vi "seq_test.vi"() -> ()   [LabVIEW 2015]
uses:
  BERTTA.dll
panel:
  out "Waveform Chart 2":dynamicdata(graph)
  out "Waveform Chart":dynamicdata(graph)
  in  "Boolean":bool
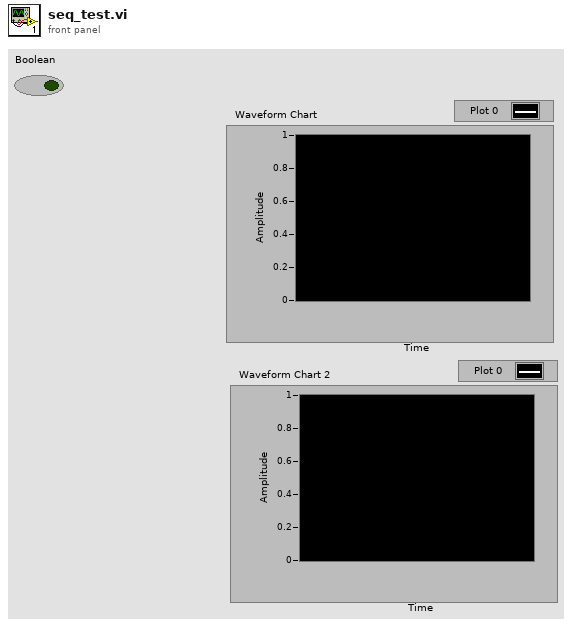
[diagram p1: front panel]
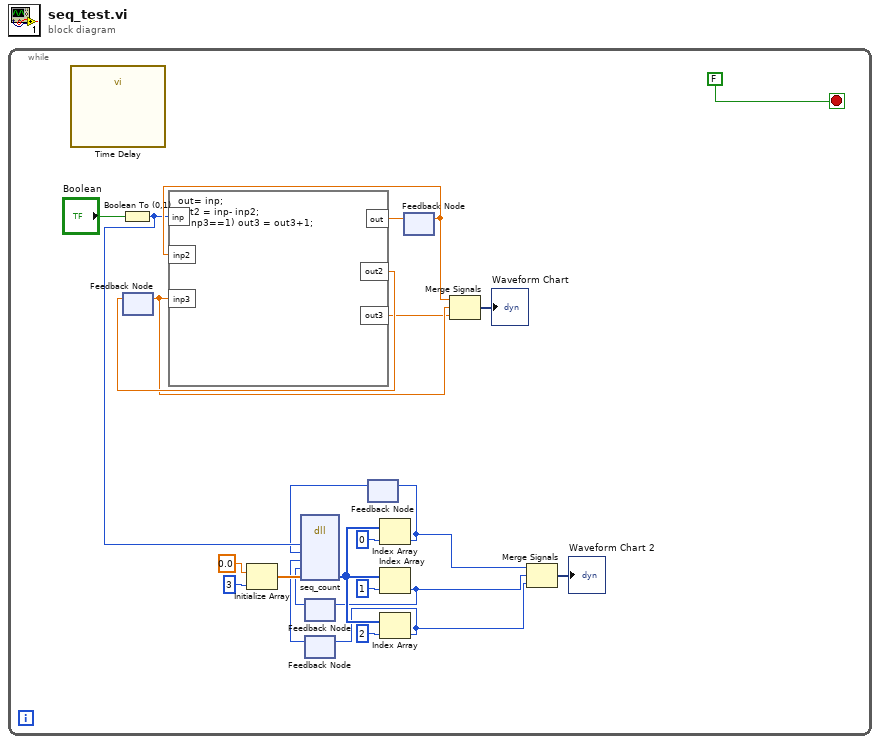
[diagram p0: block diagram]
diagram:
  n1 = while {
    stop <- FALSE stop-if-true
    n2 = call "Time Delay"() -> ()  [unwired: 11 in, 1 out]
    n3 = Boolean To (0,1)(Boolean="Boolean") -> (0, 1=w15:i16)
    n4 = feedback #1() -> (w17:dbl)  [unwired: 1 in]
    n5 = Initialize Array(0.0 ("element"), 3 ("dimension size")) -> (w14:dbl[])
    n6 = feedback #2() -> (w5:i32)  [unwired: 1 in]
    n7 = feedback #3() -> (w7:i32)  [unwired: 1 in]
    n8 = feedback #4() -> (w6:i32)  [unwired: 1 in]
    n9 = dll-call lib="C:/Users/xlaraser/Documents/Visual Studio 2017/Projects/Bertta/BERTTA/Debug/BERTTA.dll" fn="seq_count"("in1"=w15, "in2"=w6, "in3"=w7, "in4"=w5, "params"=w14) -> ("params"=w8:i32[])  [unwired: 8 in, 2 out]
    n10 = Index Array(array=w8, index=0) -> (element=w3:i32)
    n11 = feedback-in #4(w3) -> ()
    n12 = Index Array(array=w8, index=1) -> (element=w2:i32)
    n13 = feedback-in #2(w2) -> ()
    n14 = Index Array(array=w8, index=2) -> (element=w1:i32)
    n15 = feedback-in #3(w1) -> ()
    n16 = feedback #5() -> (w19:dbl)  [unwired: 1 in]
    n17 = formula code="out= inp;\nout2 = inp- inp2;\nif(inp3==1) out3 = out3+1;"("inp"=w15, "inp2"=w19, "inp3"=w17) -> ("out"=w21:dbl, "out2"=w18:dbl, "out3"=w16:dbl)
    n18 = feedback-in #1(w18) -> ()
    n19 = feedback-in #5(w21) -> ()
    n20 = Merge Signals(w19, w17, w16) -> (→"Waveform Chart":dynamicdata)
    n21 = Merge Signals(w3, w2, w1) -> (→"Waveform Chart 2":dynamicdata)
  }
